vi "Team Name.vi"(11 "MyTeam in":refnum<class "MyTeam.lvclass">) -> (2 "Team Name":string)   [LabVIEW 2020, in "SquareTeam.lvlib" / "MyTeam.lvclass"]
uses:
  MyTeam.lvclass
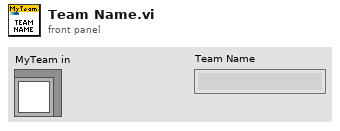
[diagram p1: front panel]
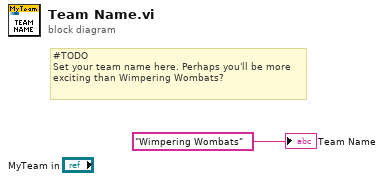
[diagram p0: block diagram]
diagram:
  # "#TODO\nSet your team name here. Perhaps you'll be more exciting than Wimpering Wombats?"
  "Team Name" <- "Wimpering Wombats" ("Team Name")
